vi "Save VI and Close Refnum.vi"(0 "VI Refnum":refnum<vi>, 11 "error in":errorcluster) -> (15 "error out":errorcluster)   [LabVIEW 2021, in "Migrator Reusables.lvlib"]
uses:
  Migrator Reusables.lvlib
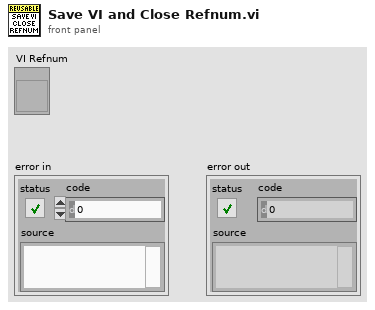
[diagram p1: front panel]
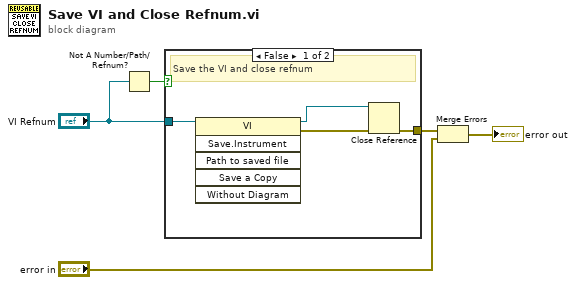
[diagram p0: block diagram]
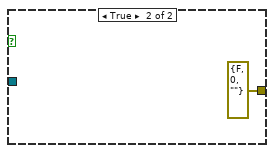
[diagram p2: hidden frame]
diagram:
  n1 = Not A Number/Path/Refnum?(number/path/refnum="VI Refnum") -> (NaN/Path/Refnum?=w3:bool)
  n2 = case shown="False" w3 {
    tunnel: [w9 errorcluster {"status"=FALSE, "code"=0, "source"=""} ("error out")] -> w5
    tunnel: "VI Refnum" -> [w6 _]
    frame False {
      # "Save the VI and close refnum"
      n3 = invoke class="VI" method="Save.Instrument"(reference=w6) -> (reference out=w7:refnum<vi>, error out=w8:errorcluster)  [unwired: 5 in, 4 out]
      n4 = Close Reference(reference=w7, error in (no error)=w8) -> (error out=w9:errorcluster)
    }
    frame True {
    }
  }
  n5 = Merge Errors(w5, "error in") -> (→"error out":errorcluster)
